vi "Change Temperature.vi"(7 "error in":errorcluster, 10 "GOTO":dbl format="%.3f") -> (0 "error out":errorcluster={"status"=TRUE, "code"=65, "source"="McP Timeout"}, 3 "Final Temperature":dbl)   [LabVIEW 2025]
doc: "McPherson 789A-3 controller Vi to control McPherson 2075 spectrometer through serial port. If running directly, you need to initialize the serial port and the spectrometer. During this process, if the scan velocity returns to be 0, the program is suspended. You need to change the velocity manually to unblock.\nAuthor: Scott Hannahs <sth@magnet.fsu.edu>\n\nThis software is licensed for use under the “MIT License\"\nCopyright (c) 2025 Scott Hannahs, sth@sth@magnet.sthnet.net\n\nPermission is hereby granted, free of charge, to any person obtaining a copy of this software and associated documentation files (the \"Software\"), to deal in the Software without restriction, including without limitation the rights to use, copy, modify, merge, publish, distribute, sublicense, and/or sell copies of the Software, and to permit persons to whom the Software is furnished to do so, subject to the following conditions: The above copyright notice and this permission notice shall be included in all copies or substantial portions of the Software.\n\nTHE SOFTWARE IS PROVIDED \"AS IS\", WITHOUT WARRANTY OF ANY KIND, EXPRESS OR IMPLIED, INCLUDING BUT NOT LIMITED TO THE WARRANTIES OF MERCHANTABILITY, FITNESS FOR A PARTICULAR PURPOSE AND NONINFRINGEMENT. IN NO EVENT SHALL THE AUTHORS OR COPYRIGHT HOLDERS BE LIABLE FOR ANY CLAIM, DAMAGES OR OTHER LIABILITY, WHETHER IN AN ACTION OF CONTRACT, TORT OR OTHERWISE, ARISING FROM, OUT OF OR IN CONNECTION WITH THE SOFTWARE OR THE USE OR OTHER DEALINGS IN THE SOFTWARE."
uses:
  Globals and TypeDefs/Type Definitions.llb/3 way Status.ctl
  Globals and TypeDefs/Error Categories.ctt
  <vilib>/Utility/error.llb/DialogType.ctl
  Globals and TypeDefs/gStatus.vi
  Globals and TypeDefs/gTemperature.vi
  Instance           8 26Saved   Change Temperature .vi
panel:
  in  "Case Constant\n(See Context Help)":bool
  in  "Reset":bool
  out "ChangeWL Status":T1(ring)
  out "CurrentPosition":dbl(knob) caption="Current Kelvin" min=550.0 max=600.0 scale=294.377..338.0 scale format="%.1f"
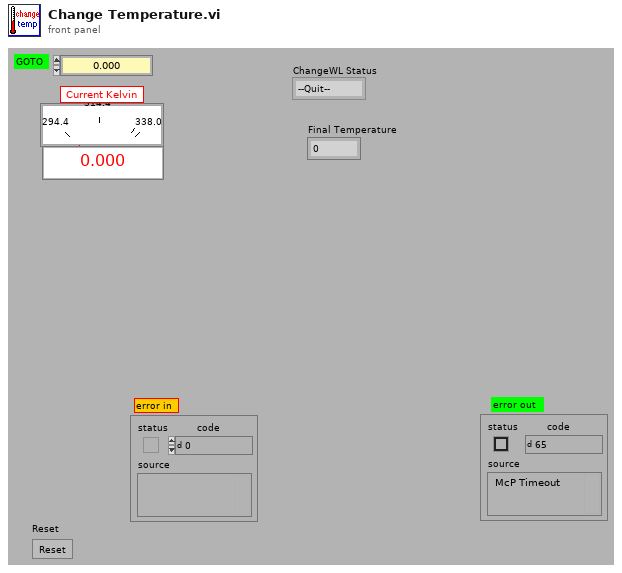
[diagram p1: front panel]
types:
  T1 = enum16{"--Quit--", "Read Initial Status", "Set New Field", "Check Field Value"}
  T2 = typedef "3 way Status.ctl" = u8
  T3 = enum16{"--Quit--", "Read Initial Status", "Set New Field", "Check Field Value", "Done"}
  T4 = enum8{"Initialization Error", "Command Error", "Parameter Error", "Overflow Error", "Time-out Error", "Misc Error", "User cancel"}
  T5 = typedef "Error Categories.ctt" = enum8{"General", "CCD-256x1024", "CCD-1340x400", "InGaAs PDA", "McPherson 2075", "Magnetic Field", "Temperature Control", "Other"}
  T6 = typedef "DialogType.ctl" = u16
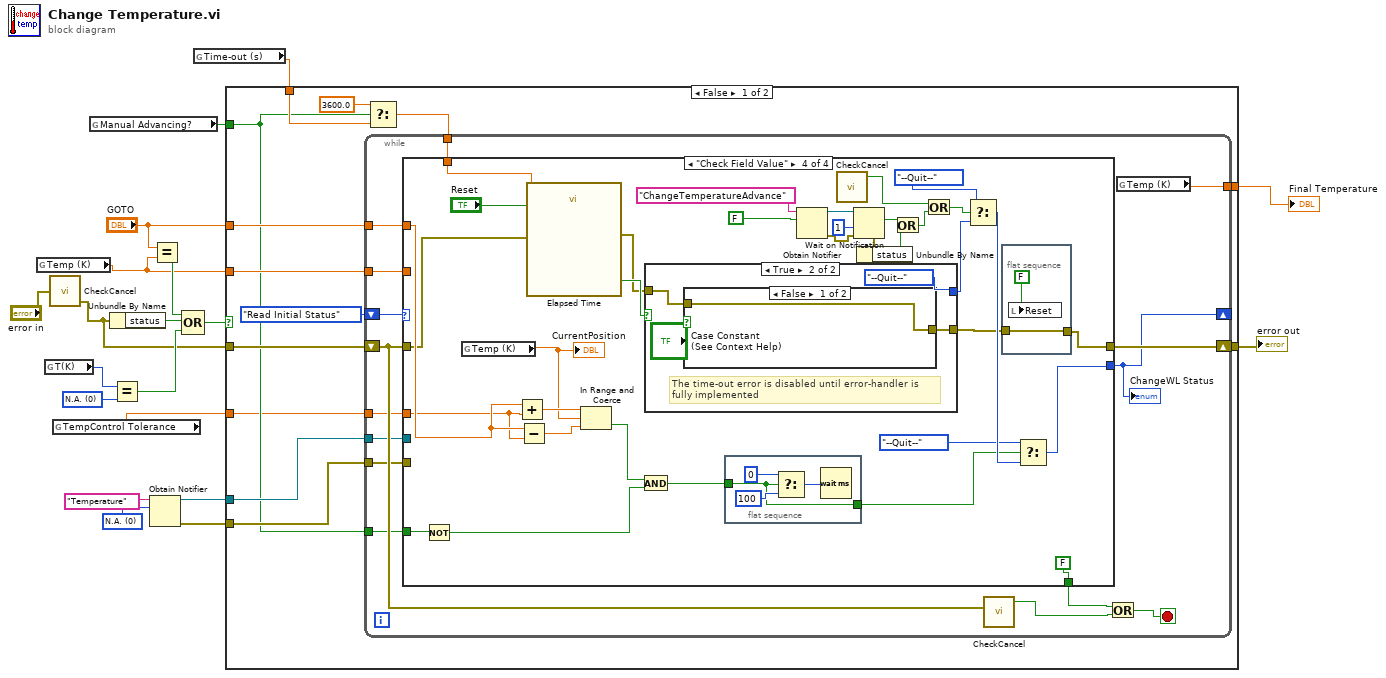
[diagram p0: block diagram]
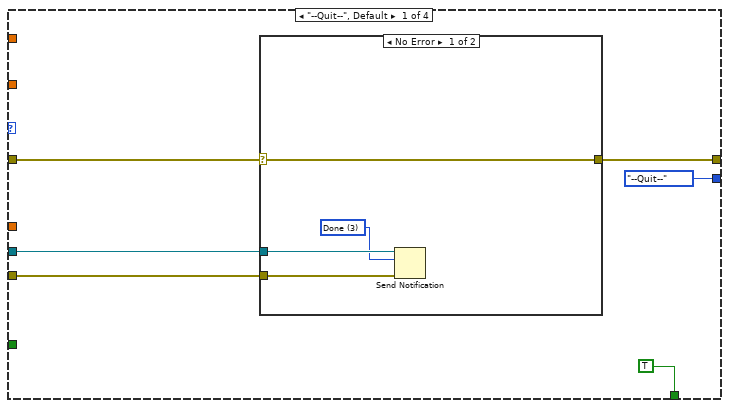
[diagram p2: hidden frame]
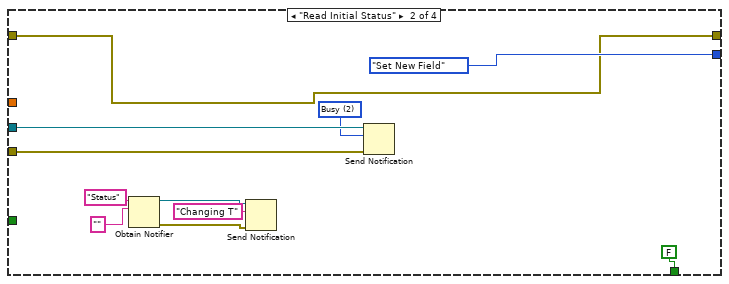
[diagram p4: hidden frame]
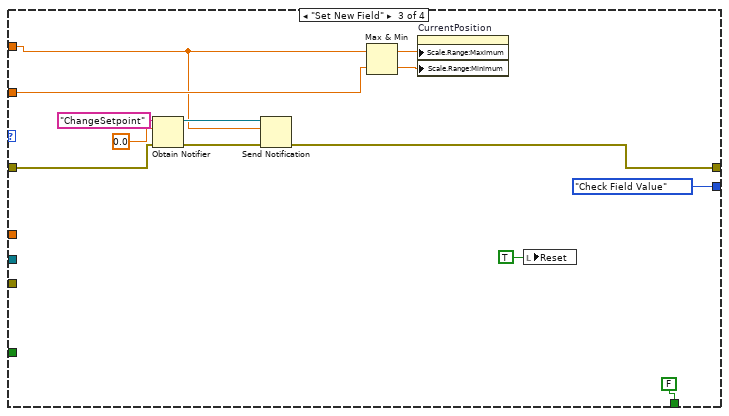
[diagram p5: hidden frame]
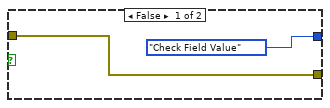
[diagram p6: hidden frame]
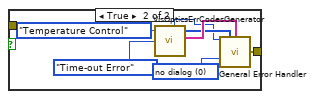
[diagram p7: hidden frame]
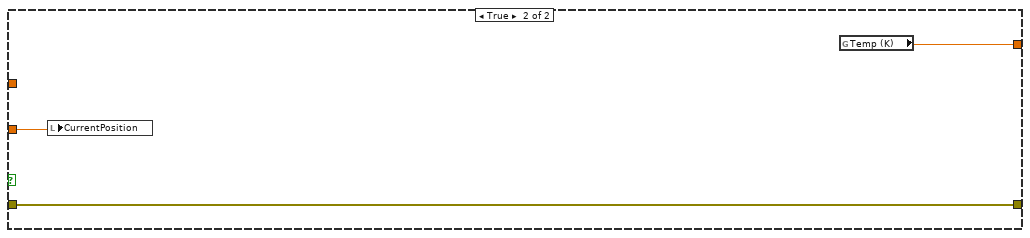
[diagram p8: hidden frame]
diagram:
  w16 = T2 0 items=["N.A.", "OK", "Busy", "Done"] ("Saving")
  w19 = T2 0 items=["N.A.", "OK", "Busy", "Done"] ("y")
  n1 = global read "gTemperature.vi" "Temp (K)"() -> (w6:dbl)
  n2 = global read "gStatus.vi" "T(K)"() -> (w18:T2)
  n3 = call "CheckCancel.vi"("error in (no error)"="error in") -> ("error out"=w2:errorcluster)  [unwired: 1 in, 1 out]
  n4 = global read "gTemperature.vi" "TempControl Tolerance"() -> (w4:dbl)
  n5 = global read "gTemperature.vi" "Manual Advancing?"() -> (w5:bool)
  n6 = Unbundle By Name(w2) -> ("status"=w11:bool)
  n7 = Equal?(x=w18, y=w19) -> (x = y?=w10:bool)
  n8 = Obtain Notifier(name (unnamed)="Temperature", notification data type=w16) -> (notifier out=w15:refnum<notifier>, error out=w14:errorcluster)  [unwired: 2 in, 1 out]
  n9 = Equal?(x="GOTO", y=w6) -> (x = y?=w12:bool)
  n10 = Compound Arithmetic op=OR(w12, w11, w10) -> (w13:bool)
  n11 = global read "gTemperature.vi" "Time-out (s)"() -> (w3:dbl)
  n12 = case shown="False" w13 {
    tunnel: w2 -> [w32 w139]
    tunnel: [w31 w139] -> w8
    tunnel: w15 -> [w30 _]
    tunnel: w14 -> [w29 _]
    tunnel: "GOTO" -> [w28 _]
    tunnel: w6 -> [w27 w138]
    tunnel: w3 -> [w24 _]
    tunnel: [w25 w137] -> w7
    tunnel: w5 -> [w21 _]
    tunnel: w4 -> [w20 _]
    frame False {
      n13 = Select(t=3600.0, s=w21, f=w24) -> (s? t:f=w23:dbl)
      n14 = while {
        shift-right: [w36] -> _
        shift-left: T3."Read Initial Status" ("ChangeField Status") -> [w47]
        shift-right: [w46] -> w31
        shift-left: w32 -> [w41]
        tunnel: w28 -> [w45]
        tunnel: w30 -> [w40]
        tunnel: w29 -> [w39]
        tunnel: w27 -> [w38]
        tunnel: w23 -> [w37]
        tunnel: [w35] -> w25
        tunnel: w21 -> [w34]
        tunnel: w20 -> [w33]
        stop <- w44 stop-if-true
        n15 = case shown="\"Check Field Value\"" w47 {
          tunnel: w41 -> [w51 w65 w76 w101]
          tunnel: [w50 w65 w72 w102] -> w46
          tunnel: w45 -> [_ _ w73 w107]
          tunnel: [T3."--Quit--" ("ChangeField Status") T3."Set New Field" ("ChangeField Status") T3."Check Field Value" ("ChangeField Status") w112] -> w36
          tunnel: [TRUE FALSE FALSE FALSE] -> w43
          tunnel: w40 -> [w49 w67 _ _]
          tunnel: w39 -> [w48 w66 _ _]
          tunnel: w38 -> [_ _ w79 _]
          tunnel: w37 -> [_ _ _ w106]
          tunnel: w34 -> [_ _ _ w88]
          tunnel: w33 -> [_ _ _ w84]
          frame "--Quit--", Default {
            n16 = case shown="No Error" w51 {
              selector: w51 -> [w54 w58]
              tunnel: [w54 w58] -> w50
              tunnel: w49 -> [w57 _]
              tunnel: w48 -> [w56 _]
              frame No Error {
                w55 = T2 3 items=["N.A.", "OK", "Busy", "Done"] ("H(T)")
                n17 = Send Notification(notification=w55, notifier=w57, error in (no error)=w56) -> ()  [unwired: 2 out]
              }
              frame Error {
              }
            }
          }
          frame "Read Initial Status" {
            w64 = T2 2 items=["N.A.", "OK", "Busy", "Done"] ("H(T)")
            n18 = Obtain Notifier(name (unnamed)="Status", notification data type="" ("Status")) -> (notifier out=w61:refnum<notifier>, error out=w60:errorcluster)  [unwired: 2 in, 1 out]
            n19 = Send Notification(notification="Changing T", notifier=w61, error in (no error)=w60) -> ()  [unwired: 2 out]
            n20 = Send Notification(notification=w64, notifier=w67, error in (no error)=w66) -> ()  [unwired: 2 out]
          }
          frame "Set New Field" {
            n21 = Obtain Notifier(name (unnamed)="ChangeSetpoint", notification data type=0.0, error in (no error)=w76) -> (notifier out=w74:refnum<notifier>, error out=w75:errorcluster)  [unwired: 1 in, 1 out]
            n22 = Send Notification(notification=w73, notifier=w74, error in (no error)=w75) -> (error out=w72:errorcluster)  [unwired: 1 out]
            n23 = Max & Min(x=w73, y=w79) -> (max(x,y)=w81:dbl, min(x,y)=w80:dbl)
            n24 = property on="CurrentPosition" class="Knob (strict)"("Scale.Range:Maximum"=w81, "Scale.Range:Minimum"=w80) -> ()  [unwired: 2 in, 2 out]
            n25 = local write "Reset"(TRUE ("Reset")) -> ()
          }
          frame "Check Field Value" {
            n26 = Not(x=w88) -> (.not. x?=w86:bool)
            n27 = global read "gTemperature.vi" "Temp (K)"() -> (w99:dbl)
            "CurrentPosition" <- w99
            n28 = Add(x=w107, y=w84) -> (x+y=w109:dbl)
            n29 = Subtract(x=w107, y=w84) -> (x-y=w108:dbl)
            n30 = call "Elapsed Time"("Time Target (s)"=w106, "Reset"="Reset", "error in (no error)"=w101) -> ("Time has Elapsed"=w105:bool, "error out"=w100:errorcluster)  [unwired: 9 in, 6 out]
            n31 = In Range and Coerce(upper limit=w109, x=w99, lower limit=w108) -> (In Range?=w87:bool)  [unwired: 1 out]
            n32 = And(x=w87, y=w86) -> (x .and. y?=w85:bool)
            n33 = case shown="True" w105 {
              tunnel: [w124 w128] -> w103
              tunnel: w100 -> [w124 w125]
              tunnel: [T3."Check Field Value" ("ChangeField Status") T3."--Quit--" ("ChangeField Status")] -> w116
              frame False {
              }
              frame True {
                # "The time-out error is disabled until error-handler is\nfully implemented"
                n34 = case shown="False" "Case Constant\n(See Context Help)" {
                  tunnel: [w129 w131] -> w128
                  tunnel: w125 -> [w129 _]
                  frame False {
                  }
                  frame True {
                    w136 = T6 0 items=["no dialog", "OK message", "continue or stop message", "OK message + warnings", "continue/stop + warnings"] ("type of dialog (OK msg:1)")
                    n35 = call "VisOpticsErrCodesGenerator.vi"("NHMFL Visible Optics Error Type"=T4."Time-out Error", "NHMFL Visible Optics Error Categories"=Error_Categories.ctt."Temperature Control") -> ("user-defined descriptions"=w135:string[], "User-defined Error Code"=w130:i32, "user-defined codes"=w134:i32[])  [unwired: 1 in, 3 out]
                    n36 = call <vilib>:"General Error Handler.vi"("[error code] (0)"=w130, "[user-defined codes]"=w134, "[user-defined descriptions]"=w135, "type of dialog (OK msg:1)"=w136) -> ("error out"=w131:errorcluster)  [unwired: 7 in, 4 out]
                  }
                }
              }
            }
            n37 = flat-sequence {
              tunnel: [w119] -> w110
              tunnel: w85 -> [w119]
              frame #0 {
                n38 = Select(t=u32 0 ("milliseconds to wait"), s=w119, f=u32 100) -> (s? t:f=w121:u32)
                n39 = Wait (ms)(milliseconds to wait=w121) -> ()  [unwired: 1 out]
              }
            }
            n40 = Obtain Notifier(name (unnamed)="ChangeTemperatureAdvance", notification data type=FALSE) -> (notifier out=w97:refnum<notifier>, error out=w94:errorcluster)  [unwired: 2 in, 1 out]
            n41 = call "CheckCancel.vi"() -> ("Cancelled"=w83:bool)  [unwired: 2 in, 1 out]
            n42 = Wait on Notification(notifier=w97, timeout in ms (-1)=1, error in (no error)=w94) -> (notification=w93:bool, error out=w92:errorcluster)  [unwired: 1 in, 2 out]
            n43 = Unbundle By Name(w92) -> ("status"=w91:bool)
            n44 = Or(x=w93, y=w91) -> (x .or. y?=w89:bool)
            n45 = Or(x=w83, y=w89) -> (x .or. y?=w90:bool)
            n46 = Select(t=T3."--Quit--" ("ChangeField Status"), s=w90, f=w116) -> (s? t:f=w114:T3)
            n47 = flat-sequence {
              tunnel: [w118] -> w102
              tunnel: w103 -> [w118]
              frame #0 {
                n48 = local write "Reset"(FALSE ("Reset")) -> ()
              }
            }
            n49 = Select(t=T3."--Quit--" ("f"), s=w110, f=w114) -> (s? t:f=w112:T3)
          }
        }
        "ChangeWL Status" <- w36
        n50 = call "CheckCancel.vi"("error in (no error)"=w41) -> ("Cancelled"=w42:bool)  [unwired: 1 in, 1 out]
        n51 = Or(x=w43, y=w42) -> (x .or. y?=w44:bool)
        n52 = global read "gTemperature.vi" "Temp (K)"() -> (w35:dbl)
      }
    }
    frame True {
      n53 = local write "CurrentPosition"(w138) -> ()
      n54 = global read "gTemperature.vi" "Temp (K)"() -> (w137:dbl)
    }
  }
  "error out" <- w8
  "Final Temperature" <- w7
